vi "Not.vi"(0 "A":bool, 7 "STOP":bool, 11 "Error in":errorcluster) -> (4 "Not":bool, 15 "Error out":errorcluster)   [LabVIEW 2020, in "Subpanel access.lvlib"]
uses:
  Subpanel access.lvlib
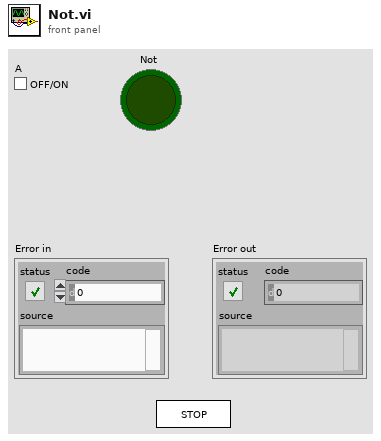
[diagram p1: front panel]
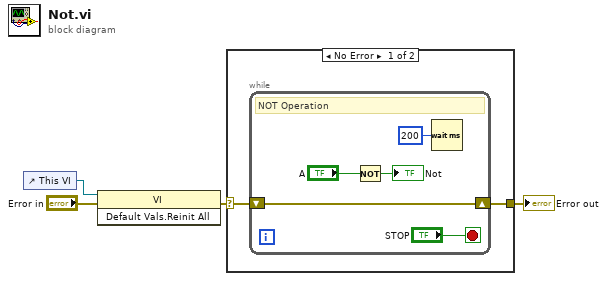
[diagram p0: block diagram]
diagram:
  n1 = control-ref of="This VI"() -> (w2:refnum<vi>)
  n2 = invoke class="VI" method="Default Vals.Reinit All"(reference=w2, error in="Error in") -> (error out=w3:errorcluster)  [unwired: 1 in, 2 out]
  n3 = case shown="No Error" w3 {
    selector: w3 -> [w5 w12]
    tunnel: [w6 w12] -> w4
    frame No Error {
      n4 = while {
        shift-right: [w11] -> w6
        shift-left: w5 -> [w11]
        stop <- "STOP" stop-if-true
        # "NOT Operation"
        n5 = Not(x="A") -> (.not. x?=→"Not":bool)
        n6 = Wait (ms)(milliseconds to wait=u32 200) -> ()  [unwired: 1 out]
      }
    }
    frame Error {
      # "Do not execute if \nerror"
    }
  }
  "Error out" <- w4
